vi "Beta Ver 1.0.vi"() -> ()   [LabVIEW 2015]
uses:
  <instrlib>/Keithley 622x LV 2009/Configure/Source/Typedefs/KE622x -- Current Range.ctl
  <instrlib>/Keithley 622x LV 2009/Configure/Source/Typedefs/KE622x -- Current Ranges.ctl
  <instrlib>/Keithley 622x LV 2009/Typedefs/KE622x -- On Off Control.ctl
  <instrlib>/Keithley 622x LV 2009/Utility/Typedefs/KE622x -- Instrument Type.ctl
  <instrlib>/Keithley 622x LV 2009/Configure/Source/Typedefs/KE622x -- Voltage Limit.ctl
  <instrlib>/Keithley 2000/Public/Configure/Configure DC Volts.vi
  <userlib>/LV-Link3/PolySubVIs/DtCreateAinChan.vi
  <userlib>/LV-Link3/PolySubVIs/DtOLReadMultipleSingle.vi
  <instrlib>/Keithley 2000/Keithley 2000.lvlib
  <instrlib>/Keithley 622x LV 2009/Keithley 622x.lvlib
panel:
  in  "Setup":u16(ring) items=["START, STOP, STEP, CONFIGURATION", "PRINCETON LOCK-IN AMP"]
  out "prev_time_const":i32
  out "prev_range":i32
  out "XTC":i32
  out "SEN":i32
  in  "Time Delay":u16(ring) items=["0.1", "1", "3", "10", "30", "60"]
  out "FILE":refnum<file>
  out "Tick":u32
  in  "MULTIPLE GRAPHS Y":u16(ring) items=["Linear", "Log"]
  in  "MULTIPLE GRAPHS X":u16(ring) items=["Linear", "Log"]
  in  "TIME GRAPH Y":u16(ring) items=["Linear", "Log"]
  in  "TIME GRAPH X":u16(ring) items=["Linear", "Log"]
  in  "Lock-In, Y":dbl=1.0
  in  "Lock-In, X":dbl=1.0
  in  "DAQ A4":dbl=1.0
  in  "DAQ A3":dbl=1.0
  in  "DAQ A2":dbl=1.0
  in  "DAQ A1":dbl=1.0
  in  "DAQ A0":dbl=1.0
  in  "2000":dbl=1.0
  in  "Current":dbl=1000.0
  in  "Display Type 3":u16(ring)=3 items=["X %", "Y %", "X Calibrated", "Y Calibrated", "Mag %", "Mag Calibrated", "Phase Degrees", "Ratio", "ADC 1", "ADC 2", "ADC 3", "ADC 4 ", "Noise %", "Noise Calibrated", "Ref Frequency", "", ""]
  in  "Display Type 2":u16(ring)=2 items=["X %", "Y %", "X Calibrated", "Y Calibrated", "Mag %", "Mag Calibrated", "Phase Degrees", "Ratio", "ADC 1", "ADC 2", "ADC 3", "ADC 4 ", "Noise %", "Noise Calibrated", "Ref Frequency", "", ""]
  out "Units 3":string
  out "Display 3":dbl format="%.3f"
  out "Units 2":string
  out "Display 2":dbl format="%.3f"
  out "DAQ A4":dbl format="%#_13g"
  out "DAQ_clust":T1
  out "DAQ A3":dbl format="%#_13g"
  out "DAQ A2":dbl format="%#_13g"
  out "DAQ A1":dbl format="%#_13g"
  out "Real stop cur":dbl format="%#_13g"
  out "Real start cur":dbl format="%#_13g"
  in  "Stop cur prefix":u16(ring)=2
  in  "Start cur prefix":u16(ring)=2
  out "MULTIPLE GRAPHS":cluster{dbl[], dbl[]}[](graph)
  in  "X-Axis":T2(ring)
  in  "Range":u8(ring)=20 items=["100nV", "200nV", "500nV", "1µV", "2µV", "5µV", "10µV", "20µV", "50µV", "100µV", "200µV", "500µV", "1mV", "2mV", "5mV", "10mV", "20mV", "50mV", "100mV", "200mV", "500mV", "1V"]
  in  "Display Type copy":u16(ring)=3 items=["X %", "Y %", "X Calibrated", "Y Calibrated", "Mag %", "Mag Calibrated", "Phase Degrees", "Ratio", "ADC 1", "ADC 2", "ADC 3", "ADC 4 ", "Noise %", "Noise Calibrated", "Ref Frequency", "", ""]
  out "Units copy":string
  out "Display copy":dbl format="%.3f"
  out "Overload":bool
  out "Display":dbl format="%.3f"
  out "Units":string
  in  "Display Type":u16(ring)=2 items=["X %", "Y %", "X Calibrated", "Y Calibrated", "Mag %", "Mag Calibrated", "Phase Degrees", "Ratio", "ADC 1", "ADC 2", "ADC 3", "ADC 4 ", "Noise %", "Noise Calibrated", "Ref Frequency", "", ""]
  in  "Time Constant":u16(ring)=7 items=["MIN", "1ms", "3ms", "10ms", "30ms", "100ms", "300ms", "1s", "3s", "10s", "30s", "100s", "300s"]
  in  "Slope":u8(ring) items=["6db/octave", "12dB/octave"]
  in  "Dynamic Reserve":u16(ring)=1 items=["High Stability", "Normal", "High Reserve"]
  in  "Auto Sensitivity":bool
  in  "Auto Measure":bool
  out "6221_error_out":errorcluster
  out "2000_error_out":errorcluster
  out "5110_error_out":errorcluster
  out "Input Mode":i32(ring) items=[" Voltage Input (A or A-B) ", "Current Input 10E6 V/A", "Current Input 10E8 V/A"]
  out "5110":refnum<visa-resource-name>
  in  "GPIB Address":i8=11 min=1 max=32 step=1
  out "DAQ A0":dbl format="%#_13g"
  out "2000":dbl format="%#_13g"
  in  "Device":string(combo)
  in  "Number \nof points":i32=10
  in  "Folder\nprename":string
  out "TIME GRAPH":cluster{dbl[], dbl[]}[](graph)
  out "T0":u32
  out "LIMIT":bool
  out "LIMIT":bool
  out "Error Code":string
  in  "Comments":string
  out "2000":refnum<visa-resource-name>
  out "6221":refnum<visa-resource-name>
  out "Step  (A)":dbl=5e-05 format="%#_3p"
  in  "Stop\ncurrent (A)":dbl=2.0 format="%#_6p"
  in  "Start \ncurrent (A)":dbl=1.0 format="%#_6p"
  in  "Check For SCPI Errors? (T)":bool=TRUE
  out "Interlock Tripped?":bool
  out "Compliance?":bool
  in  "Turn Off Output \nIf Compliance?":bool=TRUE
  in  "Turning ON/OFF\ncurrent output":T3=enum."On"
  in  "Range Selection":T4={"Auto Range?"=TRUE, "Man / Selected\nRange"=enum."2nA"}
  # "FILE CONFIGURATION"
  # "ADMIN PANEL"
  # "MULTIPLIERS"
  # "SCALES"
  # "KEITHLEY 6221 CONFIGURATION (ADMIN ONLY)"
  # "KEITHLEY DAQ CONFIGURATION (ADMIN ONLY)"
  # "PRINCETON LOCK-IN AMP (ADMIN ONLY)"
  # "I don't know what the hell it is,\njust don't touch it"
  # "INPUT CONFIGURATION"
  # "READINGS"
  # "IF ON"
  # "Compliance = Limiting output voltage\nThis switch determines if we want to switch \noff the current output if wee exceed compliance"
  # "SCALES"
  # "There is a safe switch at \nthe back of the instrument \nThis indicator shows if it is on"
  # "You have hit a damn jackpot \nby exceeding the limited voltage\nCongrats"
  # "LOCK-IN READINGS"
  # "RIGHT DISPLAY"
  # "LEFT DISPLAY"
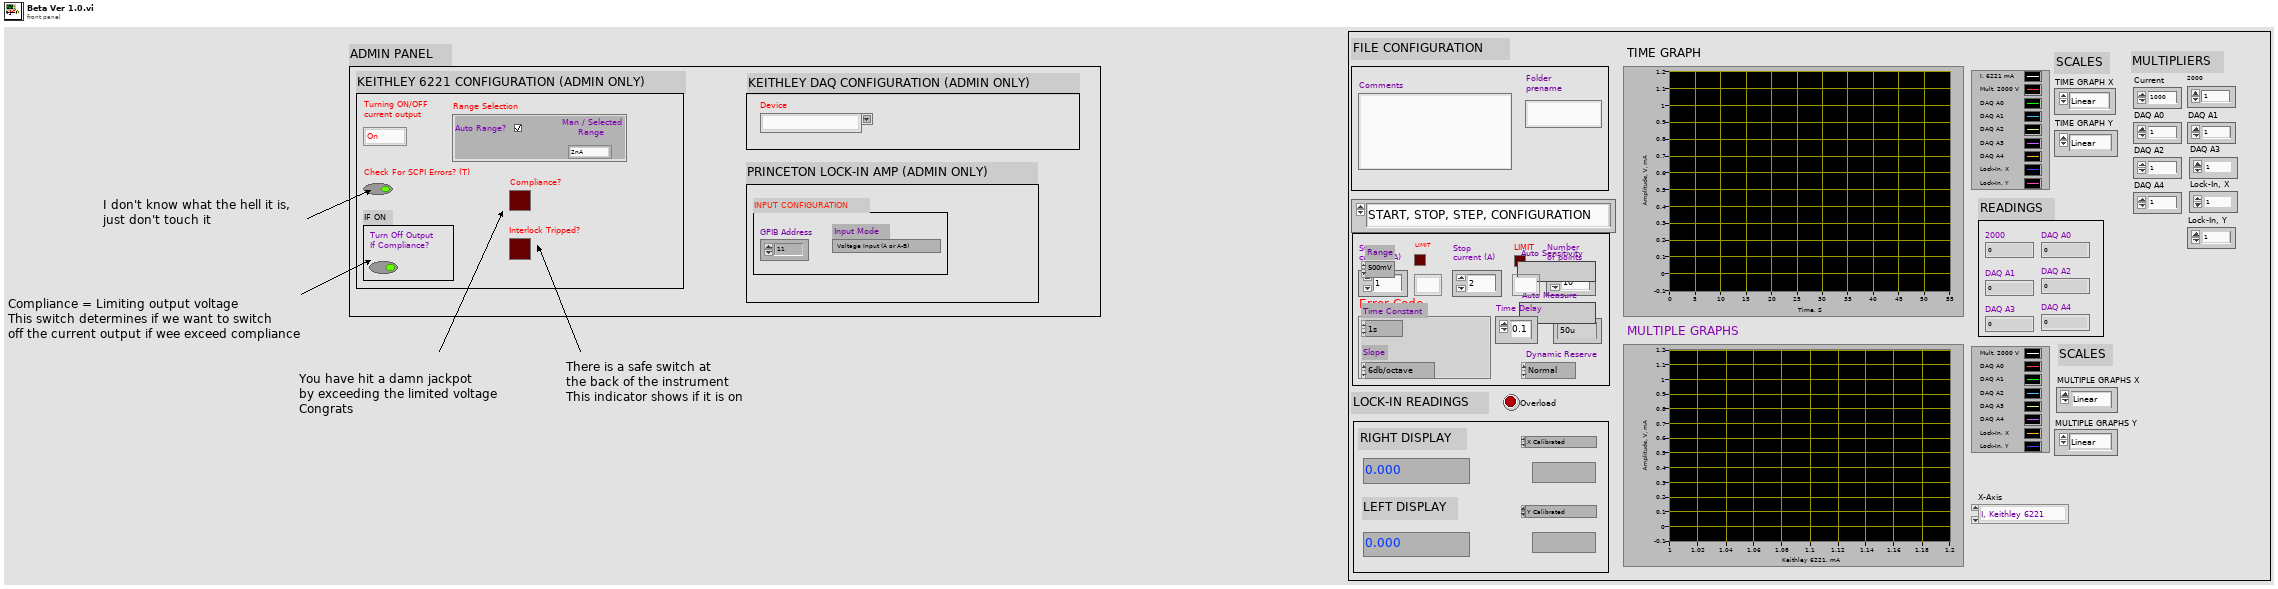
[diagram p1: front panel]
types:
  T1 = cluster{"Task out":i32, "Actual Number of Channels":u32, "error out":errorcluster}
  T2 = enum16{"I, Keithley 6221", "V, Keithley 2000", "V, Keithley DAQ A0", "V, Keithley DAQ A1", "V, Keithley DAQ A2", "V, Keithley DAQ A3", "V, Keithley DAQ A4", "V, Lock-In X", "V, Lock-In Y"}
  T3 = typedef "Keithley 622x.lvlib/KE622x -- On Off Control.ctl" = enum16{"Off", "On"}
  T4 = typedef "Keithley 622x.lvlib/KE622x -- Current Range.ctl" = cluster{"Auto Range?":bool, "Man / Selected\nRange":T5}
  T5 = typedef "Keithley 622x.lvlib/KE622x -- Current Ranges.ctl" = enum16{"2nA", "20nA", "200nA", "2uA", "20uA", "200uA", "2mA", "20mA", "100mA"}
  T6 = typedef "Keithley 622x.lvlib/KE622x -- Instrument Type.ctl" = enum16{"KE6220", "KE6221"}
  T7 = typedef "Keithley 622x.lvlib/KE622x -- Voltage Limit.ctl" = dbl
  T8 = cluster{"Task out":i32, "error out":errorcluster}
  T9 = cluster{dbl, dbl, dbl, dbl, dbl, "Measurement":dbl}
  T10 = cluster{dbl[], dbl[], dbl[], dbl[], dbl[], dbl[], dbl[], dbl[], dbl[], dbl[]}
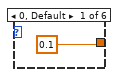
[diagram p2: hidden frame]
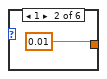
[diagram p3: hidden frame]
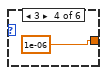
[diagram p4: hidden frame]
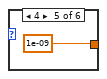
[diagram p5: hidden frame]
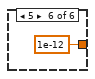
[diagram p6: hidden frame]
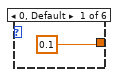
[diagram p7: hidden frame]
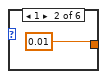
[diagram p8: hidden frame]
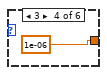
[diagram p9: hidden frame]
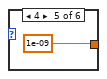
[diagram p10: hidden frame]
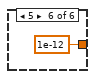
[diagram p11: hidden frame]
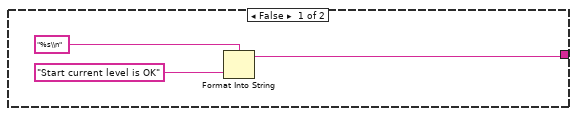
[diagram p12: hidden frame]
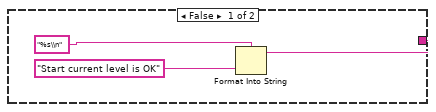
[diagram p13: hidden frame]
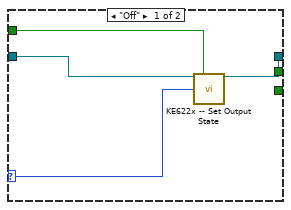
[diagram p14: hidden frame]
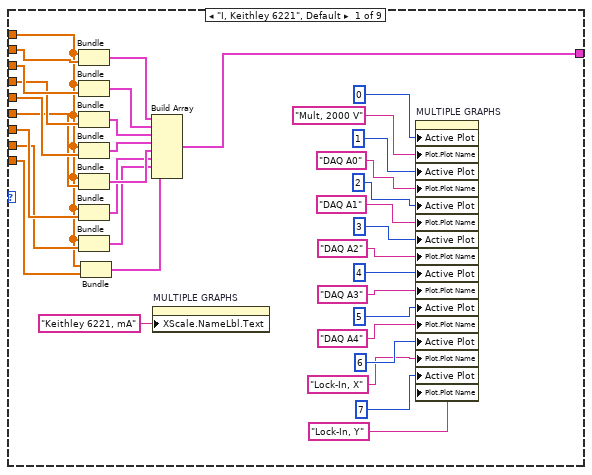
[diagram p15: hidden frame]
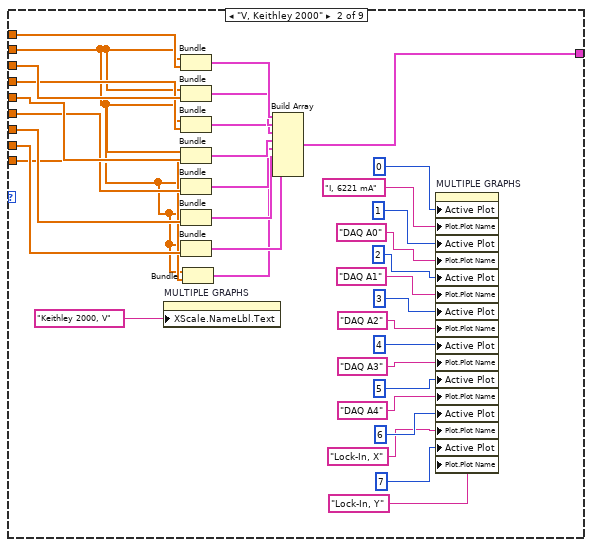
[diagram p16: hidden frame]
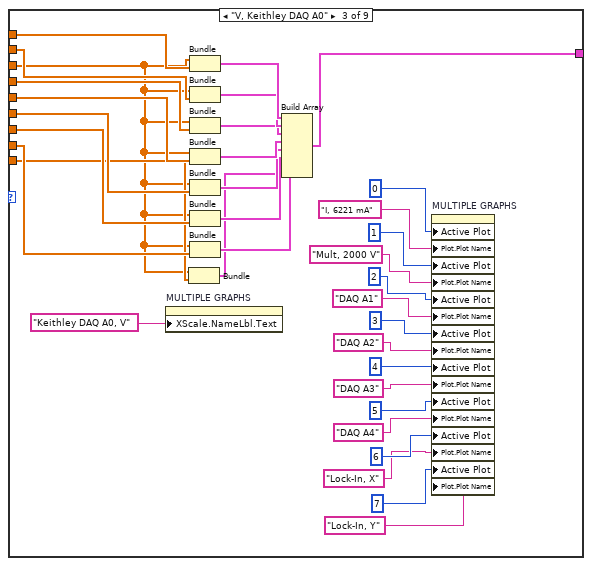
[diagram p17: hidden frame]
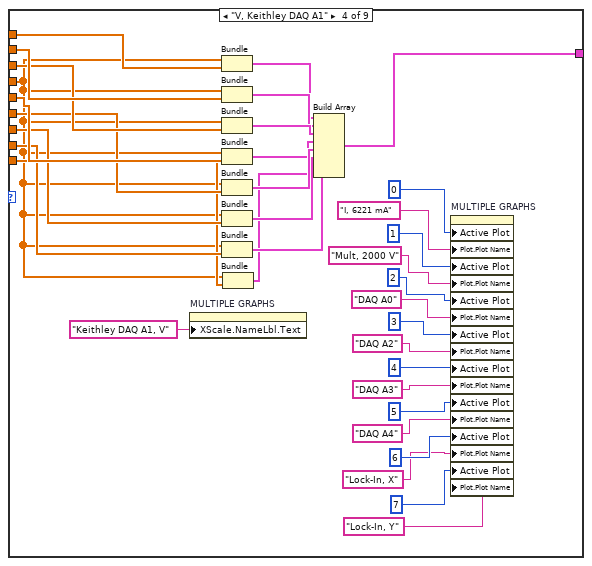
[diagram p18: hidden frame]
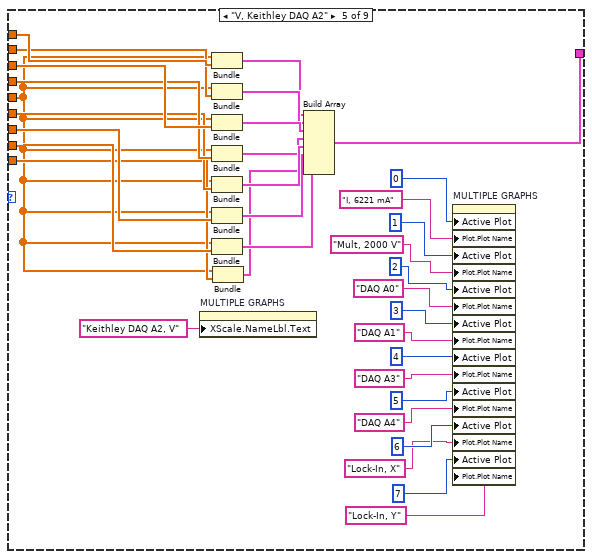
[diagram p19: hidden frame]
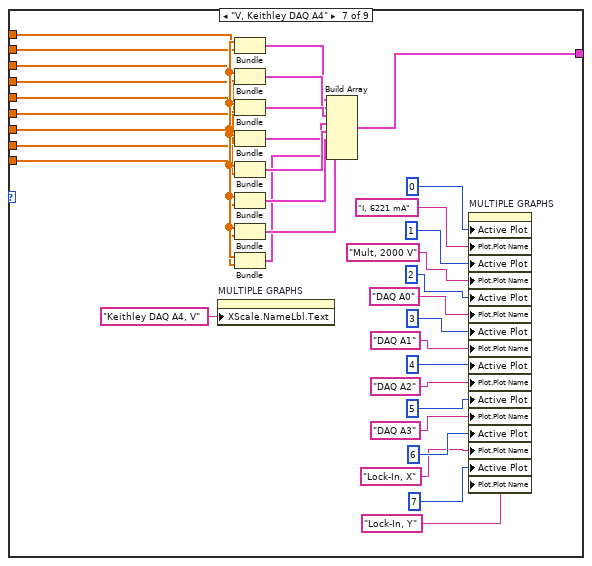
[diagram p20: hidden frame]
diagram:
  n1 = flat-sequence {
    tunnel: [w179] -> w7
    tunnel: [w178] -> w6
    tunnel: [w177] -> w5
    tunnel: [w176] -> w4
    tunnel: [w175] -> w3
    tunnel: [w174] -> w2
    tunnel: [w163] -> w1
    tunnel: w7 -> [w1070]
    tunnel: w6 -> [w1069]
    tunnel: w5 -> [w1068]
    tunnel: w4 -> [w1067]
    tunnel: w3 -> [w1066]
    tunnel: w2 -> [w1065]
    tunnel: w1 -> [w1064]
    frame #0 {
      # "File configuration"
      # "Start, Stop, Step"
      # "Initializing instruments"
      n2 = flat-sequence {
        frame #0 {
          w15 = TRUE  # reset
          w14 = FALSE  # ID query
          # "Initialize Lock-In 5110"
          # "Initialize Keithley 2000"
          # "Initialize Keithley 6221"
          n3 = call <instrlib>:"Initialize.vi"("VISA resource name"=refnum<visa-resource-name> "KEITHLEY_MULTIMETER") -> ("VISA resource name out"=w19:refnum<visa-resource-name>)  [unwired: 17 in, 1 out]
          n4 = call <instrlib>:"Initialize.vi"("VISA resource name"=refnum<visa-resource-name> "KEITHLEY_DC_AC_CURRENT_SOURCE", "Error Queue Option"=enum16{"Clear Error Queue", "Error Query"}."Clear Error Queue", "Instrument Type"=KE622x_--_Instrument_Type."KE6221") -> ("VISA resource name out"=→"6221":refnum<visa-resource-name>, "error out"=→"6221_error_out":errorcluster)  [unwired: 11 in]
          n5 = call "SR51XX Initialize"("VISA session (for class)"=refnum<visa-resource-name> "LOCK_IN_5110_PRINCETON", "Interface"=FALSE, "ID query"=w14, "GPIB Address"="GPIB Address", "reset"=w15) -> ("VISA session"=→"5110":refnum<visa-resource-name>, "error out"=→"5110_error_out":errorcluster)  [unwired: 8 in, 1 out]
          n6 = call-poly <instrlib>:"Configure Measurement.vi"("VISA resource name"=w19) -> ("VISA resource name out"=→"2000":refnum<visa-resource-name>, "error out"=→"2000_error_out":errorcluster)  [unwired: 17 in]
        }
        frame #1 {
          # "Initialize Keithley DAQ \n(getting board name)"
          n7 = call <userlib>:"DtOLGetBoardNames.vi"() -> ("Number of boards"=w24:u32)  [unwired: 9 in, 2 out]
          n8 = Initialize Array("", w24) -> (w26:string[])
          n9 = for {
            N: w24 -> [_]
            shift-right: [w32] -> w29
            shift-left: w26 -> [w33]
            i -> [w31]
            n10 = Add(x=1, y=w31) -> (x+y=w35:i32)
            n11 = call <userlib>:"DtOLGetBoardNames.vi"("Select Board"=w35) -> ("Board Name"=w30:string)  [unwired: 8 in, 2 out]
            n12 = Replace Array Subset(array=w33, new element=w30, index=w31) -> (w32:string[])
          }
          n13 = Index Array(array=w29, index=0) -> (element=w28:string)
          n14 = property on="Device" class="CmbBox"("Strings[]"=w29, "Value"=w28) -> ()  [unwired: 2 in, 2 out]
        }
        frame #2 {
          # "Putting in a loop \ninstead of \"STOP\""
          n15 = case shown="2" "Start cur prefix" {
            tunnel: [0.1 0.01 0.001 1e-06 1e-09 1e-12] -> w41
            frame 0, Default {
            }
            frame 1 {
            }
            frame 2 {
            }
            frame 3 {
            }
            frame 4 {
            }
            frame 5 {
            }
          }
          n16 = case shown="2" "Stop cur prefix" {
            tunnel: [0.1 0.01 0.001 1e-06 1e-09 1e-12] -> w39
            frame 0, Default {
            }
            frame 1 {
            }
            frame 2 {
            }
            frame 3 {
            }
            frame 4 {
            }
            frame 5 {
            }
          }
          n17 = Multiply(x=w41, y="Start \ncurrent (A)") -> (x*y=w37:dbl)
          "Real start cur" <- w37
          n18 = Multiply(x=w39, y="Stop\ncurrent (A)") -> (x*y=w36:dbl)
          "Real stop cur" <- w36
          n19 = Greater?(x=w36, y=T7 0.01) -> (0:w47:bool)
          n20 = Greater?(x=w37, y=T7 0.01) -> (0:w46:bool)
          n21 = case shown="True" w47 {
            selector: w47 -> [_ w66]
            tunnel: [w63 w69] -> w49
            frame False {
              n22 = Format Into String(format string="%s\\n", "Start current level is OK" ("false string")) -> (resulting string=w63:string)  [unwired: 2 in, 1 out]
            }
            frame True {
              n23 = flat-sequence {
                tunnel: [w71] -> w68
                tunnel: [w70] -> w67
                tunnel: w66 -> [w70]
                tunnel: [w75] -> w69
                tunnel: w68 -> [w75]
                tunnel: w67 -> [w76]
                frame #0 {
                  n24 = Format Into String(format string="%s\\n%s\\n", "Stop current level" ("String"), "exceeded the  limit: 10mA" ("input 2")) -> (resulting string=w71:string)  [unwired: 2 in, 1 out]
                }
                frame #1 {
                  n25 = while {
                    tunnel: w76 -> [w77]
                    stop <- w77 continue-if-true
                    "LIMIT" <- w77
                  }
                  n26 = property on="Error Code" class="Str"("Text.Text"=w75) -> ()  [unwired: 2 in, 2 out]
                }
              }
            }
          }
          n27 = case shown="True" w46 {
            selector: w46 -> [_ w82]
            tunnel: [w78 w84] -> w48
            frame False {
              n28 = Format Into String(format string="%s\\n", "Start current level is OK" ("false string")) -> (resulting string=w78:string)  [unwired: 2 in, 1 out]
            }
            frame True {
              n29 = flat-sequence {
                tunnel: [w86] -> w83
                tunnel: w82 -> [w85]
                tunnel: [w85] -> w81
                tunnel: [w90] -> w84
                tunnel: w83 -> [w90]
                tunnel: w81 -> [w91]
                frame #0 {
                  n30 = Format Into String(format string="%s\\n%s\\n", "Start current level" ("String"), "exceeded the limit: 10mA" ("input 2")) -> (resulting string=w86:string)  [unwired: 2 in, 1 out]
                }
                frame #1 {
                  n31 = while {
                    tunnel: w91 -> [w92]
                    stop <- w92 continue-if-true
                    "LIMIT" <- w92
                  }
                  n32 = property on="Error Code" class="Str"("Text.Text"=w90) -> ()  [unwired: 2 in, 2 out]
                }
              }
            }
          }
          n33 = Concatenate Strings(w48, w49) -> (→"Error Code":string)
        }
        frame #3 {
          # "Calculating steps by number\nof points"
          n34 = local read "Real stop cur"() -> (w96:dbl)
          n35 = local read "Real start cur"() -> (w95:dbl)
          n36 = Subtract(x=w96, y=w95) -> (x-y=w93:dbl)
          n37 = Divide(x=w93, y="Number \nof points") -> (x/y=→"Step  (A)":dbl)
        }
        frame #4 {
          # "Adding headlines"
          # "Creating folder&file"
          # "Creating comments"
          # "Writing instr params"
          n38 = local read "5110"() -> (w110:refnum<visa-resource-name>)
          n39 = local read "Real stop cur"() -> (w112:dbl)
          n40 = local read "Real start cur"() -> (w111:dbl)
          n41 = call "folder_creation.vi"("Name"="Folder\nprename") -> ("String"=w119:string)
          n42 = call "file_creation.vi"("String"=w119) -> ("refnum out"=w113:refnum<file>)
          "FILE" <- w113
          n43 = call "com_inst.vi"("Stop current"=w112, "Start current"=w111, "VISA session (for class)"=w110) -> ("XTC"=w108:i32, "SEN"=w109:i32, "concatenated string"=w107:string)
          "SEN" <- w109
          "XTC" <- w108
          n44 = Format Into String(format string="# %s\\n", initial string=w113, "Comments") -> (resulting string=w115:refnum<file>)  [unwired: 1 in, 1 out]
          n45 = property on="Time Constant" class="Ring (strict)"("Value"=w108) -> ()  [unwired: 2 in, 2 out]
          n46 = Format Into String(format string="# %s\\n", initial string=w115, w107) -> (resulting string=w114:refnum<file>)  [unwired: 1 in, 1 out]
          n47 = property on="Range" class="Ring (strict)"("Value"=w109) -> ()  [unwired: 2 in, 2 out]
          n48 = Format Into String(format string="# %-6s  %-12s %-12s %-14s %-12s %-14s %-12s %-12s %-14s%-14s\\n", initial string=w114, "t, ms" ("input 3"), "6221, A" ("input 3"), "2000, V" ("input 1"), "5110_X, V" ("input 3"), "5110_Y, V " ("input 3"), "DAQ A0, V" ("input 2"), "DAQ A1, V" ("input 2"), "DAQ A2, V" ("input 2"), "DAQ A3, V" ("input 2"), "DAQ A4, V" ("input 2")) -> ()  [unwired: 1 in, 2 out]
        }
        frame #5 {
          # "Variables"
          # "Time Intit"
          n49 = property on="SEN" class="DigNum (strict)"() -> ("Value"=→"prev_range":i32)  [unwired: 2 in, 2 out]
          n50 = property on="XTC" class="DigNum (strict)"() -> ("Value"=→"prev_time_const":i32)  [unwired: 2 in, 2 out]
          n51 = Wait Until Next ms Multiple(millisecond multiple=u32 1000) -> (millisecond timer value=→"T0":u32)
        }
      }
    }
    frame #1 {
      # "Configuring Keithley DAQ just before measuments"
      # "Configuring Keithley 6221 just before measuments"
      n52 = flat-sequence {
        tunnel: [w137] -> w127
        tunnel: [w155] -> _
        tunnel: [w157] -> _
        tunnel: w127 -> [w156]
        frame #0 {
          # "Current range \nselection check"
          # "Checking for compliance\nand interlock errors"
          n53 = local read "6221"() -> (w140:refnum<visa-resource-name>)
          n54 = call <instrlib>:"KE622x -- Set Current Range.vi"("Resource In"=w140, "Current Range In"="Range Selection", "Read Back Set Values? (T)"=FALSE) -> ("Resource Out (dupl)"=w145:refnum<visa-resource-name>)  [unwired: 10 in, 2 out]
          n55 = case shown="\"On\"" "Turning ON/OFF\ncurrent output" {
            selector: "Turning ON/OFF\ncurrent output" -> [w149 _]
            tunnel: [_ w153] -> w143
            tunnel: [_ w152] -> w144
            tunnel: "Check For SCPI Errors? (T)" -> [w148 _]
            tunnel: w145 -> [w146 w151]
            tunnel: [w147 w150] -> w137
            frame "Off" {
              n56 = call <instrlib>:"KE622x -- Set Output State.vi"("Resource In"=w146, "Check For SCPI Errors? (T)"=w148, "Output State"=w149) -> ("Resource Out (dupl)"=w147:refnum<visa-resource-name>)  [unwired: 11 in, 1 out]
            }
            frame "On" {
              n57 = call <instrlib>:"KE622x -- Turn Output On And Check For Errors.vi"("Resource In"=w151, "Turn Off Output If Compliance?"="Turn Off Output \nIf Compliance?") -> ("Resource Out (dupl)"=w150:refnum<visa-resource-name>, "Interlock Tripped?"=w153:bool, "Compliance?"=w152:bool)  [unwired: 10 in, 1 out]
            }
          }
          "Interlock Tripped?" <- w143
          "Compliance?" <- w144
        }
        frame #1 {
          # "Setting start current"
          n58 = local read "Real start cur"() -> (w155:dbl)
          n59 = Wait (ms)(milliseconds to wait=u32 100) -> ()  [unwired: 1 out]
          n60 = call <instrlib>:"KE622x -- Set Current Level.vi"("Resource In"=w156, "Current Level (A) In"=w155) -> ("Resource Out (dupl)"=w157:refnum<visa-resource-name>)  [unwired: 12 in, 1 out]
        }
      }
      n61 = flat-sequence {
        frame #0 {
          w132 = 100 items=["SingleEnded"=100, "Differential"=101] ("Channel Type")
          # "Configure the input channel"
          n62 = call-poly <userlib>:"DtOLCreateTask.vi"("Channel Type"=w132, "Range Min"=-10.0, "Range Max"=10.0, "Board Name"="Device", "Channel"="0:4" ("Channels")) -> ("Task out"=w131:i32, "Actual Number of Channels"=w130:u32, "error out"=w129:errorcluster)  [unwired: 8 in]
          n63 = Bundle("Task out"=w131, "Actual Number of Channels"=w130, "error out"=w129) -> (→"DAQ_clust":T1)  [unwired: 1 in]
        }
      }
    }
    frame #2 {
      n64 = local read "5110"() -> (w170:refnum<visa-resource-name>)
      n65 = local read "2000"() -> (w169:refnum<visa-resource-name>)
      n66 = local read "6221"() -> (w168:refnum<visa-resource-name>)
      n67 = local read "5110_error_out"() -> (w167:errorcluster)
      n68 = local read "6221_error_out"() -> (w166:errorcluster)
      n69 = local read "2000_error_out"() -> (w165:errorcluster)
      n70 = local read "DAQ_clust"() -> (w164:T1)
      n71 = while {
        shift-right: [w366] -> _
        shift-left: dbl[] [] -> [w467]
        shift-right: [w367] -> _
        shift-left: i32[] [] -> [w466]
        tunnel: w169 -> [w464]
        tunnel: w168 -> [w463]
        shift-right: [w338] -> _
        shift-left: dbl[] [] -> [w457]
        tunnel: [w456] -> w179
        tunnel: [w455] -> w178
        tunnel: [w453] -> w177
        tunnel: [w451] -> w176
        tunnel: w170 -> [w449]
        tunnel: w167 -> [w448]
        tunnel: w166 -> [w440]
        tunnel: w165 -> [w439]
        tunnel: [w414] -> w175
        tunnel: [w412] -> w174
        shift-right: [w340] -> _
        shift-left: dbl[] [] -> [w411]
        shift-right: [w341] -> _
        shift-left: dbl[] [] -> [w410]
        shift-right: [w368] -> _
        shift-left: dbl[] [] -> [w407]
        tunnel: w164 -> [w381]
        tunnel: [w380] -> w163
        shift-right: [w365] -> _
        shift-left: dbl[] [] -> [w379]
        shift-right: [w364] -> _
        shift-left: dbl[] [] -> [w378]
        shift-right: [w363] -> _
        shift-left: dbl[] [] -> [w377]
        shift-right: [w339] -> _
        shift-left: dbl[] [] -> [w343]
        i -> [w441]
        stop <- w458 stop-if-true
        # "V, DAQ A4"
        # "V, DAQ A3"
        # "V, DAQ A2"
        # "V, DAQ A1"
        # "Y-V, 5110"
        # "X-V, 5110"
        # "I, 6221"
        # "Config delay"
        # "Control subVI 5110"
        # "Read config 5110"
        # "Measurement config 5110"
        # "Time config 5110"
        # "Configuring Right Display 5110"
        # "Configuring Left Display 5110"
        # "Setting 6221 current"
        # "Delay before measuremens"
        # "Getting the data from DAQ and 2000"
        # "Changing input current"
        # "Time"
        # "V, DAQ A0"
        # "V, 2000"
        n72 = local read "T0"() -> (w465:u32)
        n73 = Quotient & Remainder(x=w441, y=10) -> (floor(x/y)=w446:i32)  [unwired: 1 out]
        n74 = Equal?(x=0, y=w441) -> (x = y?=w443:bool)
        n75 = Subtract(x=w432, y=w465) -> (x-y=w388:u32)
        n76 = Equal?(x=1, y=w446) -> (x = y?=w442:bool)
        n77 = flat-sequence {
          tunnel: w464 -> [w792]
          tunnel: [w792] -> w406
          tunnel: w463 -> [w791]
          tunnel: [w791] -> w404
          tunnel: w449 -> [w790]
          tunnel: [w790] -> w402
          tunnel: [w789] -> w400
          tunnel: w448 -> [w789]
          tunnel: w443 -> [w788]
          tunnel: [w788] -> w398
          tunnel: w442 -> [w787]
          tunnel: [w787] -> w396
          tunnel: w440 -> [w786]
          tunnel: [w786] -> w394
          tunnel: w439 -> [w785]
          tunnel: [w785] -> w392
          tunnel: [w783] -> w432
          tunnel: [w784] -> w382
          tunnel: w381 -> [w784]
          tunnel: w406 -> [w802]
          tunnel: [w802] -> w405
          tunnel: w404 -> [w801]
          tunnel: [w801] -> w403
          tunnel: w402 -> [w800]
          tunnel: [w800] -> w401
          tunnel: w400 -> [w799]
          tunnel: [w799] -> w399
          tunnel: w398 -> [w798]
          tunnel: [w798] -> w397
          tunnel: w396 -> [w797]
          tunnel: [w797] -> w395
          tunnel: w394 -> [w796]
          tunnel: [w796] -> w393
          tunnel: w392 -> [w795]
          tunnel: [w795] -> w391
          tunnel: [w794] -> w383
          tunnel: w382 -> [w794]
          tunnel: w405 -> [w819]
          tunnel: [w819] -> w431
          tunnel: w403 -> [w818]
          tunnel: [w818] -> w430
          tunnel: w401 -> [w817]
          tunnel: w399 -> [w814]
          tunnel: [w813] -> w429
          tunnel: [w812] -> w428
          tunnel: w397 -> [w811]
          tunnel: [w811] -> w427
          tunnel: w395 -> [w810]
          tunnel: w393 -> [w809]
          tunnel: [w809] -> w426
          tunnel: w391 -> [w808]
          tunnel: [w808] -> w425
          tunnel: [w807] -> w384
          tunnel: w383 -> [w807]
          tunnel: w431 -> [w844]
          tunnel: [w844] -> w239
          tunnel: w430 -> [w843]
          tunnel: [w843] -> w237
          tunnel: w429 -> [w840]
          tunnel: [w839] -> w235
          tunnel: w428 -> [w838]
          tunnel: [w837] -> w233
          tunnel: w427 -> [w835]
          tunnel: [w835] -> w231
          tunnel: w426 -> [w842]
          tunnel: [w842] -> w229
          tunnel: w425 -> [w841]
          tunnel: [w841] -> w227
          tunnel: ["Auto Measure"] -> w225
          tunnel: ["Auto Sensitivity"] -> w223
          tunnel: [w830] -> w221
          tunnel: [w828] -> w219
          tunnel: w384 -> [w828]
          tunnel: w239 -> [w858]
          tunnel: [w858] -> w238
          tunnel: w237 -> [w857]
          tunnel: [w857] -> w236
          tunnel: w235 -> [w845]
          tunnel: [w845] -> w234
          tunnel: w233 -> [w856]
          tunnel: [w856] -> w232
          tunnel: w231 -> [w855]
          tunnel: [w855] -> w230
          tunnel: w229 -> [w854]
          tunnel: [w854] -> w228
          tunnel: w227 -> [w853]
          tunnel: [w853] -> w226
          tunnel: w225 -> [w852]
          tunnel: [w852] -> w224
          tunnel: w223 -> [w851]
          tunnel: [w851] -> w222
          tunnel: w221 -> [w850]
          tunnel: [w850] -> w220
          tunnel: w219 -> [w849]
          tunnel: [w849] -> w218
          tunnel: w238 -> [w885]
          tunnel: [w885] -> w195
          tunnel: w236 -> [w884]
          tunnel: [w884] -> w197
          tunnel: w234 -> [w877]
          tunnel: w232 -> [w875]
          tunnel: [w874] -> w199
          tunnel: w230 -> [w881]
          tunnel: [w881] -> w201
          tunnel: w228 -> [w883]
          tunnel: [w883] -> w203
          tunnel: w226 -> [w882]
          tunnel: [w882] -> w205
          tunnel: w224 -> [w879]
          tunnel: [w879] -> w207
          tunnel: w222 -> [w880]
          tunnel: [w880] -> w209
          tunnel: w220 -> [w870]
          tunnel: [w870] -> w211
          tunnel: [w876] -> w213
          tunnel: ["Time Constant"] -> w215
          tunnel: ["Slope"] -> w217
          tunnel: [w868] -> w193
          tunnel: w218 -> [w868]
          tunnel: w217 -> [w901]
          tunnel: [w901] -> w216
          tunnel: w215 -> [w900]
          tunnel: [w900] -> w214
          tunnel: w213 -> [w888]
          tunnel: [w888] -> w212
          tunnel: w211 -> [w899]
          tunnel: [w899] -> w210
          tunnel: w209 -> [w898]
          tunnel: [w898] -> w208
          tunnel: w207 -> [w897]
          tunnel: [w897] -> w206
          tunnel: w205 -> [w896]
          tunnel: [w896] -> w204
          tunnel: w203 -> [w895]
          tunnel: [w895] -> w202
          tunnel: w201 -> [w894]
          tunnel: [w894] -> w200
          tunnel: w199 -> [w890]
          tunnel: [w890] -> w198
          tunnel: w197 -> [w893]
          tunnel: [w893] -> w196
          tunnel: w195 -> [w892]
          tunnel: [w892] -> w194
          tunnel: w193 -> [w891]
          tunnel: [w891] -> w192
          tunnel: [w931] -> w336
          tunnel: [w930] -> w335
          tunnel: [w916] -> w334
          tunnel: [w929] -> w333
          tunnel: [w928] -> w332
          tunnel: [w927] -> w331
          tunnel: [w926] -> w330
          tunnel: [w925] -> w329
          tunnel: [w918] -> w328
          tunnel: [w921] -> w327
          tunnel: [w919] -> w326
          tunnel: [w924] -> w325
          tunnel: w216 -> [w924]
          tunnel: w214 -> [w919]
          tunnel: w212 -> [w922]
          tunnel: w210 -> [w918]
          tunnel: w208 -> [w925]
          tunnel: w206 -> [w926]
          tunnel: w204 -> [w927]
          tunnel: w202 -> [w928]
          tunnel: w200 -> [w929]
          tunnel: w198 -> [w917]
          tunnel: w196 -> [w930]
          tunnel: w194 -> [w931]
          tunnel: [w910] -> w324
          tunnel: w192 -> [w910]
          tunnel: w336 -> [w954]
          tunnel: [w954] -> w323
          tunnel: w335 -> [w953]
          tunnel: [w953] -> w321
          tunnel: w334 -> [w945]
          tunnel: [w944] -> w319
          tunnel: w333 -> [w952]
          tunnel: [w952] -> w317
          tunnel: w332 -> [w951]
          tunnel: [w951] -> w315
          tunnel: w331 -> [w950]
          tunnel: [w950] -> w313
          tunnel: w330 -> [w949]
          tunnel: [w949] -> w311
          tunnel: w329 -> [w948]
          tunnel: [w948] -> w309
          tunnel: w328 -> [w939]
          tunnel: [w939] -> w307
          tunnel: w327 -> [w946]
          tunnel: [w943] -> w305
          tunnel: w326 -> [w941]
          tunnel: [w941] -> w303
          tunnel: w325 -> [w938]
          tunnel: [w938] -> w301
          tunnel: w324 -> [w947]
          tunnel: [w947] -> w299
          tunnel: [w934] -> w296
          tunnel: w323 -> [w977]
          tunnel: [w977] -> w322
          tunnel: w321 -> [w976]
          tunnel: [w976] -> w320
          tunnel: w319 -> [w967]
          tunnel: [w966] -> w318
          tunnel: w317 -> [w975]
          tunnel: [w975] -> w316
          tunnel: w315 -> [w974]
          tunnel: [w974] -> w314
          tunnel: w313 -> [w973]
          tunnel: [w973] -> w312
          tunnel: w311 -> [w972]
          tunnel: [w972] -> w310
          tunnel: w309 -> [w971]
          tunnel: [w971] -> w308
          tunnel: w307 -> [w962]
          tunnel: [w962] -> w306
          tunnel: w305 -> [w969]
          tunnel: [w968] -> w304
          tunnel: w303 -> [w964]
          tunnel: [w964] -> w302
          tunnel: w301 -> [w961]
          tunnel: [w961] -> w300
          tunnel: w299 -> [w970]
          tunnel: [w970] -> w298
          tunnel: [w957] -> w297
          tunnel: w322 -> [w999]
          tunnel: [w999] -> w424
          tunnel: w320 -> [w998]
          tunnel: [w998] -> w423
          tunnel: w318 -> [w985]
          tunnel: w316 -> [w997]
          tunnel: [w997] -> w422
          tunnel: w314 -> [w996]
          tunnel: [w996] -> w421
          tunnel: w312 -> [w995]
          tunnel: [w995] -> w420
          tunnel: w310 -> [w994]
          tunnel: [w994] -> w419
          tunnel: w308 -> [w993]
          tunnel: [w993] -> w418
          tunnel: w306 -> [w986]
          tunnel: w304 -> [w983]
          tunnel: [w982] -> w417
          tunnel: w302 -> [w987]
          tunnel: w300 -> [w988]
          tunnel: [w984] -> w416
          tunnel: [w981] -> w415
          tunnel: [w978] -> w385
          tunnel: w298 -> [w978]
          tunnel: [w1003] -> w462
          tunnel: w441 -> [w1011]
          tunnel: [w1007] -> w458
          tunnel: [w1001] -> w460
          tunnel: [w1009] -> w459
          tunnel: [w1006] -> w438
          tunnel: [w1005] -> w437
          tunnel: [w1004] -> w436
          tunnel: [w1002] -> w435
          tunnel: [w1001] -> w376
          tunnel: w415 -> [_]
          tunnel: w416 -> [w1004]
          tunnel: w417 -> [w1002]
          tunnel: w418 -> [_]
          tunnel: w419 -> [_]
          tunnel: w420 -> [w1006]
          tunnel: w421 -> [w1005]
          tunnel: w422 -> [_]
          tunnel: w423 -> [w1009]
          tunnel: w424 -> [w1003]
          tunnel: [w1000] -> w386
          tunnel: w385 -> [w1000]
          tunnel: w462 -> [w1024]
          tunnel: [w1024] -> w461
          tunnel: w460 -> [w1023]
          tunnel: w459 -> [w1022]
          tunnel: [w1021] -> w454
          tunnel: [w1020] -> w452
          tunnel: w438 -> [w1018]
          tunnel: w437 -> [w1019]
          tunnel: w436 -> [w1016]
          tunnel: w435 -> [w1017]
          tunnel: [w1018] -> w434
          tunnel: [w1017] -> w433
          tunnel: [w1016] -> w413
          tunnel: [w1015] -> w387
          tunnel: w386 -> [w1015]
          tunnel: [w1052] -> w380
          tunnel: [w1053] -> w412
          tunnel: [w1054] -> w414
          tunnel: [w1061] -> w450
          tunnel: [w1055] -> w351
          tunnel: [w1056] -> w451
          tunnel: [w1057] -> w453
          tunnel: [w1058] -> w455
          tunnel: [w1059] -> w456
          tunnel: [w1060] -> w350
          tunnel: [w1061] -> w346
          tunnel: [w1051] -> w349
          tunnel: [w1050] -> w348
          tunnel: [w1049] -> w347
          tunnel: w461 -> [w1048]
          tunnel: w454 -> [w1057]
          tunnel: w452 -> [w1056]
          tunnel: w434 -> [w1047]
          tunnel: w433 -> [w1054]
          tunnel: w413 -> [w1053]
          tunnel: w387 -> [w1046]
          frame #0 {
            n78 = Tick Count (ms)() -> (millisecond timer value=w783:u32)
            "Tick" <- w783
          }
          frame #1 {
            n79 = case shown="1" "Setup" {
              frame 0, Default {
                n80 = flat-sequence {
                  frame #0 {
                    w803 = FALSE ("Visible")
                    n81 = property on="Slope" class="Ring (strict)"("Visible"=w803) -> ()  [unwired: 2 in, 2 out]
                    n82 = property on="Range" class="Ring (strict)"("Visible"=w803) -> ()  [unwired: 2 in, 2 out]
                    n83 = property on="Time Constant" class="Ring (strict)"("Visible"=w803) -> ()  [unwired: 2 in, 2 out]
                    n84 = property on="Dynamic Reserve" class="Ring (strict)"("Visible"=w803) -> ()  [unwired: 2 in, 2 out]
                    n85 = property on="Auto Sensitivity" class="Bool (strict)"("Visible"=w803) -> ()  [unwired: 2 in, 2 out]
                    n86 = property on="Auto Measure" class="Bool (strict)"("Visible"=w803) -> ()  [unwired: 2 in, 2 out]
                  }
                  frame #1 {
                    w804 = TRUE ("Visible")
                    n87 = property on="Start \ncurrent (A)" class="DigNum (strict)"("Visible"=w804) -> ()  [unwired: 2 in, 2 out]
                    n88 = property on="Stop\ncurrent (A)" class="DigNum (strict)"("Visible"=w804) -> ()  [unwired: 2 in, 2 out]
                    n89 = property on="LIMIT" class="Bool (strict)"("Visible"=w804) -> ()  [unwired: 2 in, 2 out]
                    n90 = property on="LIMIT" class="Bool (strict)"("Visible"=w804) -> ()  [unwired: 2 in, 2 out]
                    n91 = property on="Start cur prefix" class="Ring (strict)"("Visible"=w804) -> ()  [unwired: 2 in, 2 out]
                    n92 = property on="Stop cur prefix" class="Ring (strict)"("Visible"=w804) -> ()  [unwired: 2 in, 2 out]
                    n93 = property on="Step  (A)" class="DigNum (strict)"("Visible"=w804) -> ()  [unwired: 2 in, 2 out]
                    n94 = property on="Number \nof points" class="DigNum (strict)"("Visible"=w804) -> ()  [unwired: 2 in, 2 out]
                    n95 = property on="Time Delay" class="Ring (strict)"("Visible"=w804) -> ()  [unwired: 2 in, 2 out]
                    n96 = property on="Error Code" class="Str"("Visible"=w804) -> ()  [unwired: 2 in, 2 out]
                  }
                }
              }
              frame 1 {
                n97 = flat-sequence {
                  frame #0 {
                    w805 = TRUE ("Visible")
                    n98 = property on="Slope" class="Ring (strict)"("Visible"=w805) -> ()  [unwired: 2 in, 2 out]
                    n99 = property on="Range" class="Ring (strict)"("Visible"=w805) -> ()  [unwired: 2 in, 2 out]
                    n100 = property on="Time Constant" class="Ring (strict)"("Visible"=w805) -> ()  [unwired: 2 in, 2 out]
                    n101 = property on="Dynamic Reserve" class="Ring (strict)"("Visible"=w805) -> ()  [unwired: 2 in, 2 out]
                    n102 = property on="Auto Sensitivity" class="Bool (strict)"("Visible"=w805) -> ()  [unwired: 2 in, 2 out]
                    n103 = property on="Auto Measure" class="Bool (strict)"("Visible"=w805) -> ()  [unwired: 2 in, 2 out]
                  }
                  frame #1 {
                    w806 = FALSE ("Visible")
                    n104 = property on="Start \ncurrent (A)" class="DigNum (strict)"("Visible"=w806) -> ()  [unwired: 2 in, 2 out]
                    n105 = property on="Stop\ncurrent (A)" class="DigNum (strict)"("Visible"=w806) -> ()  [unwired: 2 in, 2 out]
                    n106 = property on="LIMIT" class="Bool (strict)"("Visible"=w806) -> ()  [unwired: 2 in, 2 out]
                    n107 = property on="LIMIT" class="Bool (strict)"("Visible"=w806) -> ()  [unwired: 2 in, 2 out]
                    n108 = property on="Start cur prefix" class="Ring (strict)"("Visible"=w806) -> ()  [unwired: 2 in, 2 out]
                    n109 = property on="Stop cur prefix" class="Ring (strict)"("Visible"=w806) -> ()  [unwired: 2 in, 2 out]
                    n110 = property on="Step  (A)" class="DigNum (strict)"("Visible"=w806) -> ()  [unwired: 2 in, 2 out]
                    n111 = property on="Number \nof points" class="DigNum (strict)"("Visible"=w806) -> ()  [unwired: 2 in, 2 out]
                    n112 = property on="Time Delay" class="Ring (strict)"("Visible"=w806) -> ()  [unwired: 2 in, 2 out]
                    n113 = property on="Error Code" class="Str"("Visible"=w806) -> ()  [unwired: 2 in, 2 out]
                  }
                }
              }
            }
          }
          frame #2 {
            n114 = case shown="False" w810 {
              tunnel: w817 -> [w821 w826]
              tunnel: [w820 w824] -> w816
              tunnel: [w821 w823] -> w815
              tunnel: w814 -> [w820 w822]
              frame False {
              }
              frame True {
                n115 = call "SR51XX Read Preamp Input Mode"("VISA session (for class)"=w826, "error in (no error)"=w822) -> ("VISA session"=w823:refnum<visa-resource-name>, "Input Mode"=w825:i32, "error out"=w824:errorcluster)  [unwired: 15 in]
                n116 = local write "Input Mode"(w825) -> ()
              }
            }
            n117 = call "SR51XX Configure Signal Channel Input"("VISA session (for class)"=w815, "error in (no error)"=w816, "Update"=w811) -> ("VISA session"=w813:refnum<visa-resource-name>, "error out"=w812:errorcluster)  [unwired: 15 in]
          }
          frame #3 {
            n118 = local read "Input Mode"() -> (w836:i32)
            n119 = call "SR51XX Configure Sensitivity"("VISA session (for class)"=w840, "Input Mode"=w836, "Range"="Range", "error in (no error)"=w838, "Auto Sensitivity"="Auto Sensitivity", "Auto Measure"="Auto Measure", "Update"=w835) -> ("Range Annotations Out[]"=w829:string[], "VISA session"=w839:refnum<visa-resource-name>, "Auto Sensitivity out"=w832:bool, "Auto Measure out"=w831:bool, "Range Out"=w830:u8, "error out"=w837:errorcluster)  [unwired: 7 in]
            n120 = property on="Range" class="Ring (strict)"("Strings []"=w829) -> ()  [unwired: 2 in, 2 out]
            n121 = local write "Auto Sensitivity"(w832) -> ()
            n122 = local write "Auto Measure"(w831) -> ()
            n123 = local write "Range"(w830) -> ()
          }
          frame #4 {
            n124 = property on="prev_range" class="DigNum (strict)"() -> ("Value"=w847:i32)  [unwired: 2 in, 2 out]
            n125 = property on="Range" class="Ring (strict)"() -> ("Value"=w846:u8)  [unwired: 2 in, 2 out]
            n126 = Equal?(x=w846, y=w847) -> (x = y?=w848:bool)
            n127 = case shown="False" w848 {
              tunnel: w845 -> [w859 _]
              frame False {
                n128 = flat-sequence {
                  tunnel: w859 -> [w861]
                  frame #0 {
                    n129 = property on="Range" class="Ring (strict)"() -> ("Value"=w860:u8)  [unwired: 2 in, 2 out]
                    n130 = property on="prev_range" class="DigNum (strict)"("Value"=w860) -> ()  [unwired: 2 in, 2 out]
                  }
                  frame #1 {
                    n131 = call "read_sense.vi"("VISA session (for class)"=w861) -> ("sense"=w863:string)
                    n132 = Concatenate Strings("Sensitivity: " ("string"), w863) -> (w862:string)
                    n133 = local read "FILE"() -> (w866:refnum<file>)
                    n134 = Format Into String(format string="# %-s\\n", initial string=w866, w862) -> ()  [unwired: 1 in, 2 out]
                  }
                }
              }
              frame True {
              }
            }
          }
          frame #5 {
            n135 = Or(x=w880, y=w879) -> (x .or. y?=w878:bool)
            n136 = call "SR51XX Configure Output Channels - Slope, TC and Dyn Reserve"("VISA session (for class)"=w877, "Time Constant"="Time Constant", "Slope"="Slope", "Check TC"=w878, "Dynamic Reserve"="Dynamic Reserve", "error in (no error)"=w875, "Range"=w870, "Update"=w881) -> ("VISA session"=w876:refnum<visa-resource-name>, "Slope Out"=w871:u8, "Time Constant Out"=w872:u16, "error out"=w874:errorcluster)  [unwired: 8 in]
            n137 = local write "Slope"(w871) -> ()
            n138 = local write "Time Constant"(w872) -> ()
          }
          frame #6 {
            n139 = property on="prev_time_const" class="DigNum (strict)"() -> ("Value"=w887:i32)  [unwired: 2 in, 2 out]
            n140 = property on="Time Constant" class="Ring (strict)"() -> ("Value"=w886:u16)  [unwired: 2 in, 2 out]
            n141 = Equal?(x=w886, y=w887) -> (x = y?=w889:bool)
            n142 = case shown="False" w889 {
              tunnel: w888 -> [w902 _]
              frame False {
                n143 = flat-sequence {
                  tunnel: w902 -> [w904]
                  frame #0 {
                    n144 = property on="Time Constant" class="Ring (strict)"() -> ("Value"=w903:u16)  [unwired: 2 in, 2 out]
                    n145 = property on="prev_time_const" class="DigNum (strict)"("Value"=w903) -> ()  [unwired: 2 in, 2 out]
                  }
                  frame #1 {
                    n146 = call "read_time_const.vi"("VISA session (for class)"=w904) -> ("time_const"=w905:string)
                    n147 = Concatenate Strings("Time Constant: " ("string"), w905) -> (w906:string)
                    n148 = local read "FILE"() -> (w909:refnum<file>)
                    n149 = Format Into String(format string="# %-s\\n", initial string=w909, w906) -> ()  [unwired: 1 in, 2 out]
                  }
                }
              }
              frame True {
              }
            }
          }
          frame #7 {
            n150 = local read "Input Mode"() -> (w923:i32)
            n151 = call "SR5110 Read Output"("VISA session (for class)"=w922, "Input Mode"=w923, "Time Constant"=w919, "Display Type"="Display Type", "Range"=w918, "error in (no error)"=w917, "Slope"=w924) -> ("Units"=→"Units":string, "Display Precision"=w915:i32, "Display"=→"Display":dbl, "VISA session"=w921:refnum<visa-resource-name>, "Available Display Types Out"=w914:string[], "Overload"=→"Overload":bool, "error out"=w916:errorcluster)  [unwired: 4 in, 2 out]
            n152 = property on="Display Type" class="Ring (strict)"("Strings []"=w914) -> ()  [unwired: 2 in, 2 out]
            n153 = property on="Display" class="DigNum (strict)"("Precision"=w915) -> ()  [unwired: 2 in, 2 out]
          }
          frame #8 {
            n154 = local read "Input Mode"() -> (w942:i32)
            n155 = call "SR5110 Read Output"("VISA session (for class)"=w946, "Input Mode"=w942, "Time Constant"=w941, "Display Type"="Display Type 2", "Range"=w939, "error in (no error)"=w945, "Slope"=w938) -> ("Units"=w932:string, "Display Precision"=w936:i32, "Display"=w933:dbl, "VISA session"=w943:refnum<visa-resource-name>, "Available Display Types Out"=w937:string[], "error out"=w944:errorcluster)  [unwired: 4 in, 3 out]
            "Display 2" <- w933
            "Units 2" <- w932
            n156 = call "pref_to_num.vi"("string"=w932) -> ("Numeric"=w935:dbl)
            n157 = property on="Display Type 2" class="Ring (strict)"("Strings []"=w937) -> ()  [unwired: 2 in, 2 out]
            n158 = property on="Display 2" class="DigNum (strict)"("Precision"=w936) -> ()  [unwired: 2 in, 2 out]
            n159 = Multiply(x=w935, y=w933) -> (x*y=w934:dbl)
          }
          frame #9 {
            n160 = local read "Input Mode"() -> (w965:i32)
            n161 = call "SR5110 Read Output"("VISA session (for class)"=w969, "Input Mode"=w965, "Time Constant"=w964, "Display Type"="Display Type 3", "Range"=w962, "error in (no error)"=w967, "Slope"=w961) -> ("Units"=w956:string, "Display Precision"=w960:i32, "Display"=w955:dbl, "VISA session"=w968:refnum<visa-resource-name>, "Available Display Types Out"=w959:string[], "error out"=w966:errorcluster)  [unwired: 4 in, 3 out]
            "Display 3" <- w955
            "Units 3" <- w956
            n162 = property on="Display 3" class="DigNum (strict)"("Precision"=w960) -> ()  [unwired: 2 in, 2 out]
            n163 = call "pref_to_num.vi"("string"=w956) -> ("Numeric"=w958:dbl)
            n164 = property on="Display Type 3" class="Ring (strict)"("Strings []"=w959) -> ()  [unwired: 2 in, 2 out]
            n165 = Multiply(x=w958, y=w955) -> (x*y=w957:dbl)
          }
          frame #10 {
            n166 = local read "Input Mode"() -> (w992:i32)
            n167 = call "SR5110 Read Output"("VISA session (for class)"=w983, "Input Mode"=w992, "Time Constant"=w987, "Display Type"="Display Type copy", "Range"=w986, "error in (no error)"=w985, "Slope"=w988) -> ("Units"=→"Units copy":string, "Display Precision"=w989:i32, "Display"=→"Display copy":dbl, "VISA session"=w982:refnum<visa-resource-name>, "Reference Unlock"=w981:bool, "Available Display Types Out"=w990:string[], "error out"=w984:errorcluster)  [unwired: 4 in, 2 out]
            n168 = property on="Display Type copy" class="Ring (strict)"("Strings []"=w990) -> ()  [unwired: 2 in, 2 out]
            n169 = property on="Display copy" class="DigNum (strict)"("Precision"=w989) -> ()  [unwired: 2 in, 2 out]
          }
          frame #11 {
            n170 = local read "Step  (A)"() -> (w1012:dbl)
            n171 = local read "Real start cur"() -> (w1013:dbl)
            n172 = Multiply(x=w1012, y=w1011) -> (x*y=w1010:dbl)
            n173 = Add(x=w1013, y=w1010) -> (x+y=w1001:dbl)
            n174 = local read "Real stop cur"() -> (w1008:dbl)
            n175 = Greater Or Equal?(x=w1001, y=w1008) -> (x >= y?=w1007:bool)
          }
          frame #12 {
            n176 = call <instrlib>:"KE622x -- Set Current Level.vi"("Resource In"=w1022, "Current Level (A) In"=w1023, "error in (no error)"=w1019) -> ("Resource Out (dupl)"=w1020:refnum<visa-resource-name>, "error out"=w1021:errorcluster)  [unwired: 11 in]
            n177 = Wait Until Next ms Multiple(millisecond multiple=u32 50) -> ()  [unwired: 1 out]
          }
          frame #13 {
            n178 = Unbundle(w1046) -> ("Task out"=w1045:i32, "Actual Number of Channels"=w1043:u32, "error out"=w1044:errorcluster)
            n179 = call <instrlib>:"Data Read Single.vi"("VISA resource name"=w1048, "error in (no error)"=w1047) -> ("VISA resource name out"=w1058:refnum<visa-resource-name>, "Measurement"=w1061:dbl, "error out"=w1059:errorcluster)  [unwired: 13 in, 2 out]
            n180 = call-poly <userlib>:"DtOLRead.vi"("Number Chan to Read"=w1043, "error in (no error)"=w1044, "Task in"=w1045) -> ("error out"=w1041:errorcluster, "2D Data out"=w1040:dbl[][], "Task out"=w1042:i32)  [unwired: 4 in, 2 out]
            n181 = Index Array(array=w1040, index (row) #1=0 ("index (row)"), index (row) #2=1 ("index (row)"), index (row) #3=2 ("index (row)"), index (row) #4=3 ("index (row)"), index (row) #5=4 ("index (row)")) -> (element #1=w1039:dbl[], element #2=w1033:dbl[], element #3=w1032:dbl[], element #4=w1031:dbl[], element #5=w1030:dbl[])  [unwired: 5 in]
            n182 = Index Array(array=w1030, index=0) -> (element=w1049:dbl)
            n183 = Index Array(array=w1039, index=0) -> (element=w1055:dbl)
            n184 = Index Array(array=w1033, index=0) -> (element=w1060:dbl)
            n185 = Index Array(array=w1032, index=0) -> (element=w1051:dbl)
            n186 = Index Array(array=w1031, index=0) -> (element=w1050:dbl)
            n187 = Bundle("Task out"=w1042, "error out"=w1041) -> (w1052:T8)  [unwired: 1 in]
          }
        }
        n188 = Divide(x=w388, y=u32 1000) -> (x/y=w389:dbl)
        n189 = local read "FILE"() -> (w243:refnum<file>)
        n190 = Build Array (concatenate)(w466, w389) -> (w374:dbl[])
        n191 = property on="TIME GRAPH" class="XYGraph (strict)"("XScale.Mapping Mode"="TIME GRAPH X", "YScale.Mapping Mode"="TIME GRAPH Y") -> ()  [unwired: 2 in, 2 out]
        n192 = property on="MULTIPLE GRAPHS" class="XYGraph (strict)"("XScale.Mapping Mode"="MULTIPLE GRAPHS X", "YScale.Mapping Mode"="MULTIPLE GRAPHS Y") -> ()  [unwired: 2 in, 2 out]
        n193 = Bundle(w376, w296, w297) -> (w249:cluster{dbl, dbl, dbl})  [unwired: 1 in]
        n194 = Unbundle(w249) -> (w293:dbl, w259:dbl, w254:dbl)
        n195 = Unbundle(w249) -> (w191:dbl, w190:dbl, w189:dbl)
        n196 = Multiply(x=w293, y="Current") -> (x*y=w292:dbl)
        n197 = Multiply(x=w254, y="Lock-In, Y") -> (x*y=w255:dbl)
        n198 = Multiply(x=w259, y="Lock-In, X") -> (x*y=w260:dbl)
        n199 = Build Array (concatenate)(w407, w292) -> (w375:dbl[])
        n200 = Build Array (concatenate)(w411, w260) -> (w345:dbl[])
        n201 = Build Array (concatenate)(w410, w255) -> (w344:dbl[])
        n202 = Bundle(w351, w350, w349, w348, w347, "Measurement"=w346) -> (w352:T9)  [unwired: 1 in]
        n203 = Unbundle(w352) -> (w285:dbl, w279:dbl, w274:dbl, w269:dbl, w264:dbl, "Measurement"=w288:dbl)
        n204 = Unbundle(w352) -> (w187:dbl, w186:dbl, w185:dbl, w184:dbl, w183:dbl, "Measurement"=w188:dbl)
        n205 = Format Into String(format string="%08d  %8.2e %12g %14.5e %12.4e %12.4e  %12.4e %12.4e  %12.4e  %12g \\n", initial string=w243, w388, w191, w188, w190, w189, w187, w186, w185, w184, w183) -> ()  [unwired: 1 in, 2 out]
        n206 = Multiply(x=w288, y="2000") -> (x*y=w286:dbl)
        n207 = Multiply(x=w279, y="DAQ A1") -> (x*y=w280:dbl)
        n208 = Multiply(x=w285, y="DAQ A0") -> (x*y=w284:dbl)
        n209 = Multiply(x="DAQ A2", y=w274) -> (x*y=w275:dbl)
        n210 = Multiply(x=w264, y="DAQ A4") -> (x*y=w265:dbl)
        n211 = Multiply(x=w269, y="DAQ A3") -> (x*y=w270:dbl)
        n212 = Build Array (concatenate)(w467, w286) -> (w373:dbl[])
        n213 = Build Array (concatenate)(w379, w284) -> (w372:dbl[])
        n214 = Build Array (concatenate)(w378, w280) -> (w371:dbl[])
        n215 = Build Array (concatenate)(w377, w275) -> (w370:dbl[])
        n216 = Build Array (concatenate)(w457, w270) -> (w369:dbl[])
        n217 = Build Array (concatenate)(w343, w265) -> (w342:dbl[])
        n218 = Bundle(w375, w374, w373, w372, w371, w370, w369, w342, w345, w344) -> (w362:T10)  [unwired: 1 in]
        n219 = Unbundle(w362) -> (w294:dbl[], w252:dbl[], w291:dbl[], w282:dbl[], w277:dbl[], w272:dbl[], w267:dbl[], w261:dbl[], w257:dbl[], w251:dbl[])
        n220 = Bundle(w252, w294) -> (w295:cluster{dbl[], dbl[]})  [unwired: 1 in]
        n221 = Bundle(w252, w291) -> (w290:cluster{dbl[], dbl[]})  [unwired: 1 in]
        n222 = Bundle(w252, w282) -> (w281:cluster{dbl[], dbl[]})  [unwired: 1 in]
        n223 = Bundle(w252, w277) -> (w276:cluster{dbl[], dbl[]})  [unwired: 1 in]
        n224 = Bundle(w252, w267) -> (w266:cluster{dbl[], dbl[]})  [unwired: 1 in]
        n225 = Bundle(w252, w272) -> (w271:cluster{dbl[], dbl[]})  [unwired: 1 in]
        n226 = Bundle(w252, w261) -> (w262:cluster{dbl[], dbl[]})  [unwired: 1 in]
        n227 = Bundle(w252, w257) -> (w256:cluster{dbl[], dbl[]})  [unwired: 1 in]
        n228 = Bundle(w252, w251) -> (w250:cluster{dbl[], dbl[]})  [unwired: 1 in]
        n229 = Build Array(w295, w290, w281, w276, w271, w266, w262, w256, w250) -> (→"TIME GRAPH":cluster{dbl[], dbl[]}[])
        n230 = Unbundle(w362) -> (w361:dbl[], w360:dbl[], w359:dbl[], w358:dbl[], w357:dbl[], w356:dbl[], w355:dbl[], w354:dbl[], w337:dbl[])  [unwired: 1 out]
        n231 = case shown="\"V, Keithley DAQ A3\"" "X-Axis" {
          tunnel: [w487 w529 w564 w592 w634 w669 w704 w729 w764] -> w353
          tunnel: w361 -> [w484 w528 w563 w599 w633 w668 w702 w737 w772]
          tunnel: w360 -> [w501 w519 w562 w598 w632 w667 w701 w736 w771]
          tunnel: w359 -> [w500 w527 w554 w597 w631 w666 w700 w735 w770]
          tunnel: w358 -> [w499 w526 w561 w589 w630 w665 w699 w734 w769]
          tunnel: w357 -> [w498 w525 w560 w596 w624 w664 w698 w733 w768]
          tunnel: w356 -> [w497 w524 w559 w595 w629 w659 w697 w732 w767]
          tunnel: w355 -> [w496 w523 w558 w594 w628 w663 w703 w731 w766]
          tunnel: w354 -> [w495 w522 w557 w593 w627 w662 w696 w738 w765]
          tunnel: w337 -> [w485 w520 w555 w590 w625 w660 w695 w730 w773]
          frame "I, Keithley 6221", Default {
            n232 = Bundle(w484, w501) -> (w494:cluster{dbl[], dbl[]})  [unwired: 1 in]
            n233 = Bundle(w484, w500) -> (w493:cluster{dbl[], dbl[]})  [unwired: 1 in]
            n234 = Bundle(w484, w499) -> (w492:cluster{dbl[], dbl[]})  [unwired: 1 in]
            n235 = Bundle(w484, w498) -> (w491:cluster{dbl[], dbl[]})  [unwired: 1 in]
            n236 = Bundle(w484, w497) -> (w490:cluster{dbl[], dbl[]})  [unwired: 1 in]
            n237 = Bundle(w484, w496) -> (w489:cluster{dbl[], dbl[]})  [unwired: 1 in]
            n238 = Bundle(w484, w495) -> (w488:cluster{dbl[], dbl[]})  [unwired: 1 in]
            n239 = Bundle(w484, w485) -> (w486:cluster{dbl[], dbl[]})  [unwired: 1 in]
            n240 = Build Array(w494, w493, w492, w491, w490, w489, w488, w486) -> (w487:cluster{dbl[], dbl[]}[])
            n241 = property on="MULTIPLE GRAPHS" class="XYGraph (strict)"("XScale.NameLbl.Text"="Keithley 6221, mA" ("X Scale.Name Label.Text")) -> ()  [unwired: 2 in, 2 out]
            n242 = property on="MULTIPLE GRAPHS" class="XYGraph (strict)"("Active Plot"=u32 0, "Plot.Plot Name"="Mult, 2000 V", "Active Plot"=u32 1, "Plot.Plot Name"="DAQ A0", "Active Plot"=u32 2, "Plot.Plot Name"="DAQ A1", "Active Plot"=u32 3, "Plot.Plot Name"="DAQ A2", "Active Plot"=u32 4, "Plot.Plot Name"="DAQ A3", "Active Plot"=u32 5, "Plot.Plot Name"="DAQ A4", "Active Plot"=u32 6, "Plot.Plot Name"="Lock-In, X", "Active Plot"=u32 7, "Plot.Plot Name"="Lock-In, Y") -> ()  [unwired: 2 in, 2 out]
          }
          frame "V, Keithley 2000" {
            n243 = property on="MULTIPLE GRAPHS" class="XYGraph (strict)"("XScale.NameLbl.Text"="Keithley 2000, V" ("X Scale.Name Label.Text")) -> ()  [unwired: 2 in, 2 out]
            n244 = Bundle(w519, w528) -> (w536:cluster{dbl[], dbl[]})  [unwired: 1 in]
            n245 = Bundle(w519, w527) -> (w535:cluster{dbl[], dbl[]})  [unwired: 1 in]
            n246 = Bundle(w519, w526) -> (w534:cluster{dbl[], dbl[]})  [unwired: 1 in]
            n247 = Bundle(w519, w525) -> (w533:cluster{dbl[], dbl[]})  [unwired: 1 in]
            n248 = Bundle(w519, w524) -> (w532:cluster{dbl[], dbl[]})  [unwired: 1 in]
            n249 = Bundle(w519, w523) -> (w531:cluster{dbl[], dbl[]})  [unwired: 1 in]
            n250 = Bundle(w519, w522) -> (w530:cluster{dbl[], dbl[]})  [unwired: 1 in]
            n251 = Bundle(w519, w520) -> (w521:cluster{dbl[], dbl[]})  [unwired: 1 in]
            n252 = Build Array(w536, w535, w534, w533, w532, w531, w530, w521) -> (w529:cluster{dbl[], dbl[]}[])
            n253 = property on="MULTIPLE GRAPHS" class="XYGraph (strict)"("Active Plot"=u32 0, "Plot.Plot Name"="I, 6221 mA", "Active Plot"=u32 1, "Plot.Plot Name"="DAQ A0", "Active Plot"=u32 2, "Plot.Plot Name"="DAQ A1", "Active Plot"=u32 3, "Plot.Plot Name"="DAQ A2", "Active Plot"=u32 4, "Plot.Plot Name"="DAQ A3", "Active Plot"=u32 5, "Plot.Plot Name"="DAQ A4", "Active Plot"=u32 6, "Plot.Plot Name"="Lock-In, X", "Active Plot"=u32 7, "Plot.Plot Name"="Lock-In, Y") -> ()  [unwired: 2 in, 2 out]
          }
          frame "V, Keithley DAQ A0" {
            n254 = property on="MULTIPLE GRAPHS" class="XYGraph (strict)"("XScale.NameLbl.Text"="Keithley DAQ A0, V" ("X Scale.Name Label.Text")) -> ()  [unwired: 2 in, 2 out]
            n255 = Bundle(w554, w555) -> (w556:cluster{dbl[], dbl[]})  [unwired: 1 in]
            n256 = Bundle(w554, w563) -> (w571:cluster{dbl[], dbl[]})  [unwired: 1 in]
            n257 = Bundle(w554, w562) -> (w570:cluster{dbl[], dbl[]})  [unwired: 1 in]
            n258 = Bundle(w554, w561) -> (w569:cluster{dbl[], dbl[]})  [unwired: 1 in]
            n259 = Bundle(w554, w560) -> (w568:cluster{dbl[], dbl[]})  [unwired: 1 in]
            n260 = Bundle(w554, w559) -> (w567:cluster{dbl[], dbl[]})  [unwired: 1 in]
            n261 = Bundle(w554, w558) -> (w566:cluster{dbl[], dbl[]})  [unwired: 1 in]
            n262 = Bundle(w554, w557) -> (w565:cluster{dbl[], dbl[]})  [unwired: 1 in]
            n263 = Build Array(w571, w570, w569, w568, w567, w566, w565, w556) -> (w564:cluster{dbl[], dbl[]}[])
            n264 = property on="MULTIPLE GRAPHS" class="XYGraph (strict)"("Active Plot"=u32 0, "Plot.Plot Name"="I, 6221 mA", "Active Plot"=u32 1, "Plot.Plot Name"="Mult, 2000 V", "Active Plot"=u32 2, "Plot.Plot Name"="DAQ A1", "Active Plot"=u32 3, "Plot.Plot Name"="DAQ A2", "Active Plot"=u32 4, "Plot.Plot Name"="DAQ A3", "Active Plot"=u32 5, "Plot.Plot Name"="DAQ A4", "Active Plot"=u32 6, "Plot.Plot Name"="Lock-In, X", "Active Plot"=u32 7, "Plot.Plot Name"="Lock-In, Y") -> ()  [unwired: 2 in, 2 out]
          }
          frame "V, Keithley DAQ A1" {
            n265 = property on="MULTIPLE GRAPHS" class="XYGraph (strict)"("XScale.NameLbl.Text"="Keithley DAQ A1, V" ("X Scale.Name Label.Text")) -> ()  [unwired: 2 in, 2 out]
            n266 = Bundle(w589, w599) -> (w601:cluster{dbl[], dbl[]})  [unwired: 1 in]
            n267 = Bundle(w589, w598) -> (w602:cluster{dbl[], dbl[]})  [unwired: 1 in]
            n268 = Bundle(w589, w597) -> (w603:cluster{dbl[], dbl[]})  [unwired: 1 in]
            n269 = Bundle(w589, w596) -> (w604:cluster{dbl[], dbl[]})  [unwired: 1 in]
            n270 = Bundle(w589, w595) -> (w605:cluster{dbl[], dbl[]})  [unwired: 1 in]
            n271 = Bundle(w589, w594) -> (w606:cluster{dbl[], dbl[]})  [unwired: 1 in]
            n272 = Bundle(w589, w593) -> (w607:cluster{dbl[], dbl[]})  [unwired: 1 in]
            n273 = Bundle(w589, w590) -> (w591:cluster{dbl[], dbl[]})  [unwired: 1 in]
            n274 = Build Array(w601, w602, w603, w604, w605, w606, w607, w591) -> (w592:cluster{dbl[], dbl[]}[])
            n275 = property on="MULTIPLE GRAPHS" class="XYGraph (strict)"("Active Plot"=u32 0, "Plot.Plot Name"="I, 6221 mA", "Active Plot"=u32 1, "Plot.Plot Name"="Mult, 2000 V", "Active Plot"=u32 2, "Plot.Plot Name"="DAQ A0", "Active Plot"=u32 3, "Plot.Plot Name"="DAQ A2", "Active Plot"=u32 4, "Plot.Plot Name"="DAQ A3", "Active Plot"=u32 5, "Plot.Plot Name"="DAQ A4", "Active Plot"=u32 6, "Plot.Plot Name"="Lock-In, X", "Active Plot"=u32 7, "Plot.Plot Name"="Lock-In, Y") -> ()  [unwired: 2 in, 2 out]
          }
          frame "V, Keithley DAQ A2" {
            n276 = property on="MULTIPLE GRAPHS" class="XYGraph (strict)"("XScale.NameLbl.Text"="Keithley DAQ A2, V" ("X Scale.Name Label.Text")) -> ()  [unwired: 2 in, 2 out]
            n277 = Bundle(w624, w633) -> (w635:cluster{dbl[], dbl[]})  [unwired: 1 in]
            n278 = Bundle(w624, w632) -> (w636:cluster{dbl[], dbl[]})  [unwired: 1 in]
            n279 = Bundle(w624, w631) -> (w637:cluster{dbl[], dbl[]})  [unwired: 1 in]
            n280 = Bundle(w624, w630) -> (w638:cluster{dbl[], dbl[]})  [unwired: 1 in]
            n281 = Bundle(w624, w629) -> (w639:cluster{dbl[], dbl[]})  [unwired: 1 in]
            n282 = Bundle(w624, w628) -> (w640:cluster{dbl[], dbl[]})  [unwired: 1 in]
            n283 = Bundle(w624, w627) -> (w641:cluster{dbl[], dbl[]})  [unwired: 1 in]
            n284 = Bundle(w624, w625) -> (w626:cluster{dbl[], dbl[]})  [unwired: 1 in]
            n285 = Build Array(w635, w636, w637, w638, w639, w640, w641, w626) -> (w634:cluster{dbl[], dbl[]}[])
            n286 = property on="MULTIPLE GRAPHS" class="XYGraph (strict)"("Active Plot"=u32 0, "Plot.Plot Name"="I, 6221 mA", "Active Plot"=u32 1, "Plot.Plot Name"="Mult, 2000 V", "Active Plot"=u32 2, "Plot.Plot Name"="DAQ A0", "Active Plot"=u32 3, "Plot.Plot Name"="DAQ A1", "Active Plot"=u32 4, "Plot.Plot Name"="DAQ A3", "Active Plot"=u32 5, "Plot.Plot Name"="DAQ A4", "Active Plot"=u32 6, "Plot.Plot Name"="Lock-In, X", "Active Plot"=u32 7, "Plot.Plot Name"="Lock-In, Y") -> ()  [unwired: 2 in, 2 out]
          }
          frame "V, Keithley DAQ A3" {
            n287 = property on="MULTIPLE GRAPHS" class="XYGraph (strict)"("XScale.NameLbl.Text"="Keithley DAQ A3, V" ("X Scale.Name Label.Text")) -> ()  [unwired: 2 in, 2 out]
            n288 = Bundle(w659, w668) -> (w670:cluster{dbl[], dbl[]})  [unwired: 1 in]
            n289 = Bundle(w659, w667) -> (w671:cluster{dbl[], dbl[]})  [unwired: 1 in]
            n290 = Bundle(w659, w666) -> (w672:cluster{dbl[], dbl[]})  [unwired: 1 in]
            n291 = Bundle(w659, w665) -> (w673:cluster{dbl[], dbl[]})  [unwired: 1 in]
            n292 = Bundle(w659, w664) -> (w674:cluster{dbl[], dbl[]})  [unwired: 1 in]
            n293 = Bundle(w659, w663) -> (w675:cluster{dbl[], dbl[]})  [unwired: 1 in]
            n294 = Bundle(w659, w662) -> (w676:cluster{dbl[], dbl[]})  [unwired: 1 in]
            n295 = Bundle(w659, w660) -> (w661:cluster{dbl[], dbl[]})  [unwired: 1 in]
            n296 = Build Array(w670, w671, w672, w673, w674, w675, w676, w661) -> (w669:cluster{dbl[], dbl[]}[])
            n297 = property on="MULTIPLE GRAPHS" class="XYGraph (strict)"("Active Plot"=u32 0, "Plot.Plot Name"="I, 6221 mA", "Active Plot"=u32 1, "Plot.Plot Name"="Mult, 2000 V", "Active Plot"=u32 2, "Plot.Plot Name"="DAQ A0", "Active Plot"=u32 3, "Plot.Plot Name"="DAQ A1", "Active Plot"=u32 4, "Plot.Plot Name"="DAQ A2", "Active Plot"=u32 5, "Plot.Plot Name"="DAQ A4", "Active Plot"=u32 6, "Plot.Plot Name"="Lock-In, X", "Active Plot"=u32 7, "Plot.Plot Name"="Lock-In,Y") -> ()  [unwired: 2 in, 2 out]
          }
          frame "V, Keithley DAQ A4" {
            n298 = property on="MULTIPLE GRAPHS" class="XYGraph (strict)"("XScale.NameLbl.Text"="Keithley DAQ A4, V" ("X Scale.Name Label.Text")) -> ()  [unwired: 2 in, 2 out]
            n299 = Bundle(w703, w702) -> (w706:cluster{dbl[], dbl[]})  [unwired: 1 in]
            n300 = Bundle(w703, w701) -> (w707:cluster{dbl[], dbl[]})  [unwired: 1 in]
            n301 = Bundle(w703, w700) -> (w708:cluster{dbl[], dbl[]})  [unwired: 1 in]
            n302 = Bundle(w703, w699) -> (w709:cluster{dbl[], dbl[]})  [unwired: 1 in]
            n303 = Bundle(w703, w698) -> (w710:cluster{dbl[], dbl[]})  [unwired: 1 in]
            n304 = Bundle(w703, w697) -> (w711:cluster{dbl[], dbl[]})  [unwired: 1 in]
            n305 = Bundle(w703, w696) -> (w712:cluster{dbl[], dbl[]})  [unwired: 1 in]
            n306 = Bundle(w703, w695) -> (w705:cluster{dbl[], dbl[]})  [unwired: 1 in]
            n307 = Build Array(w706, w707, w708, w709, w710, w711, w712, w705) -> (w704:cluster{dbl[], dbl[]}[])
            n308 = property on="MULTIPLE GRAPHS" class="XYGraph (strict)"("Active Plot"=u32 0, "Plot.Plot Name"="I, 6221 mA", "Active Plot"=u32 1, "Plot.Plot Name"="Mult, 2000 V", "Active Plot"=u32 2, "Plot.Plot Name"="DAQ A0", "Active Plot"=u32 3, "Plot.Plot Name"="DAQ A1", "Active Plot"=u32 4, "Plot.Plot Name"="DAQ A2", "Active Plot"=u32 5, "Plot.Plot Name"="DAQ A3", "Active Plot"=u32 6, "Plot.Plot Name"="Lock-In, X", "Active Plot"=u32 7, "Plot.Plot Name"="Lock-In, Y") -> ()  [unwired: 2 in, 2 out]
          }
          frame "V, Lock-In X" {
            n309 = property on="MULTIPLE GRAPHS" class="XYGraph (strict)"("XScale.NameLbl.Text"="Lock-In X, V" ("X Scale.Name Label.Text")) -> ()  [unwired: 2 in, 2 out]
            n310 = Bundle(w738, w737) -> (w740:cluster{dbl[], dbl[]})  [unwired: 1 in]
            n311 = Bundle(w738, w736) -> (w741:cluster{dbl[], dbl[]})  [unwired: 1 in]
            n312 = Bundle(w738, w735) -> (w742:cluster{dbl[], dbl[]})  [unwired: 1 in]
            n313 = Bundle(w738, w734) -> (w743:cluster{dbl[], dbl[]})  [unwired: 1 in]
            n314 = Bundle(w738, w733) -> (w744:cluster{dbl[], dbl[]})  [unwired: 1 in]
            n315 = Bundle(w738, w732) -> (w745:cluster{dbl[], dbl[]})  [unwired: 1 in]
            n316 = Bundle(w738, w731) -> (w746:cluster{dbl[], dbl[]})  [unwired: 1 in]
            n317 = Bundle(w738, w730) -> (w739:cluster{dbl[], dbl[]})  [unwired: 1 in]
            n318 = Build Array(w740, w741, w742, w743, w744, w745, w746, w739) -> (w729:cluster{dbl[], dbl[]}[])
            n319 = property on="MULTIPLE GRAPHS" class="XYGraph (strict)"("Active Plot"=u32 0, "Plot.Plot Name"="I, 6221 mA", "Active Plot"=u32 1, "Plot.Plot Name"="Mult, 2000 V", "Active Plot"=u32 2, "Plot.Plot Name"="DAQ A0", "Active Plot"=u32 3, "Plot.Plot Name"="DAQ A1", "Active Plot"=u32 4, "Plot.Plot Name"="DAQ A2", "Active Plot"=u32 5, "Plot.Plot Name"="DAQ A3", "Active Plot"=u32 6, "Plot.Plot Name"="DAQ A4", "Active Plot"=u32 7, "Plot.Plot Name"="Lock-In, Y") -> ()  [unwired: 2 in, 2 out]
          }
          frame "V, Lock-In Y" {
            n320 = property on="MULTIPLE GRAPHS" class="XYGraph (strict)"("XScale.NameLbl.Text"="Lock-In Y, V" ("X Scale.Name Label.Text")) -> ()  [unwired: 2 in, 2 out]
            n321 = Bundle(w773, w772) -> (w781:cluster{dbl[], dbl[]})  [unwired: 1 in]
            n322 = Bundle(w773, w771) -> (w780:cluster{dbl[], dbl[]})  [unwired: 1 in]
            n323 = Bundle(w773, w770) -> (w779:cluster{dbl[], dbl[]})  [unwired: 1 in]
            n324 = Bundle(w773, w769) -> (w778:cluster{dbl[], dbl[]})  [unwired: 1 in]
            n325 = Bundle(w773, w768) -> (w777:cluster{dbl[], dbl[]})  [unwired: 1 in]
            n326 = Bundle(w773, w767) -> (w776:cluster{dbl[], dbl[]})  [unwired: 1 in]
            n327 = Bundle(w773, w766) -> (w775:cluster{dbl[], dbl[]})  [unwired: 1 in]
            n328 = Bundle(w773, w765) -> (w774:cluster{dbl[], dbl[]})  [unwired: 1 in]
            n329 = Build Array(w781, w780, w779, w778, w777, w776, w775, w774) -> (w764:cluster{dbl[], dbl[]}[])
            n330 = property on="MULTIPLE GRAPHS" class="XYGraph (strict)"("Active Plot"=u32 0, "Plot.Plot Name"="I, 6221 mA", "Active Plot"=u32 1, "Plot.Plot Name"="Mult, 2000 V", "Active Plot"=u32 2, "Plot.Plot Name"="DAQ A0", "Active Plot"=u32 3, "Plot.Plot Name"="DAQ A1", "Active Plot"=u32 4, "Plot.Plot Name"="DAQ A2", "Active Plot"=u32 5, "Plot.Plot Name"="DAQ A3", "Active Plot"=u32 6, "Plot.Plot Name"="DAQ A4", "Active Plot"=u32 7, "Plot.Plot Name"="Lock-In, X") -> ()  [unwired: 2 in, 2 out]
          }
        }
        "MULTIPLE GRAPHS" <- w353
        n331 = Unbundle(w362) -> (w368:dbl[], w367:dbl[], w366:dbl[], w365:dbl[], w364:dbl[], w363:dbl[], w338:dbl[], w339:dbl[], w340:dbl[], w341:dbl[])
        n332 = Multiply(x="Time Delay", y=u16 1000) -> (x*y=w242:u16)
        n333 = Wait Until Next ms Multiple(millisecond multiple=w242) -> ()  [unwired: 1 out]
        "2000" <- w450
        "DAQ A0" <- w351
        "DAQ A1" <- w350
        "DAQ A2" <- w349
        "DAQ A3" <- w348
        "DAQ A4" <- w347
      }
    }
    frame #3 {
      # "Closing instrumental \nconnections"
      n334 = flat-sequence {
        frame #0 {
          w1072 = TRUE ("Visible")
          n335 = property on="Slope" class="Ring (strict)"("Visible"=w1072) -> ()  [unwired: 2 in, 2 out]
          n336 = property on="Range" class="Ring (strict)"("Visible"=w1072) -> ()  [unwired: 2 in, 2 out]
          n337 = property on="Time Constant" class="Ring (strict)"("Visible"=w1072) -> ()  [unwired: 2 in, 2 out]
          n338 = property on="Dynamic Reserve" class="Ring (strict)"("Visible"=w1072) -> ()  [unwired: 2 in, 2 out]
          n339 = property on="Auto Sensitivity" class="Bool (strict)"("Visible"=w1072) -> ()  [unwired: 2 in, 2 out]
          n340 = property on="Auto Measure" class="Bool (strict)"("Visible"=w1072) -> ()  [unwired: 2 in, 2 out]
        }
        frame #1 {
          w1073 = TRUE ("Visible")
          n341 = property on="Start \ncurrent (A)" class="DigNum (strict)"("Visible"=w1073) -> ()  [unwired: 2 in, 2 out]
          n342 = property on="Stop\ncurrent (A)" class="DigNum (strict)"("Visible"=w1073) -> ()  [unwired: 2 in, 2 out]
          n343 = property on="LIMIT" class="Bool (strict)"("Visible"=w1073) -> ()  [unwired: 2 in, 2 out]
          n344 = property on="LIMIT" class="Bool (strict)"("Visible"=w1073) -> ()  [unwired: 2 in, 2 out]
          n345 = property on="Start cur prefix" class="Ring (strict)"("Visible"=w1073) -> ()  [unwired: 2 in, 2 out]
          n346 = property on="Stop cur prefix" class="Ring (strict)"("Visible"=w1073) -> ()  [unwired: 2 in, 2 out]
          n347 = property on="Step  (A)" class="DigNum (strict)"("Visible"=w1073) -> ()  [unwired: 2 in, 2 out]
          n348 = property on="Number \nof points" class="DigNum (strict)"("Visible"=w1073) -> ()  [unwired: 2 in, 2 out]
          n349 = property on="Time Delay" class="Ring (strict)"("Visible"=w1073) -> ()  [unwired: 2 in, 2 out]
          n350 = property on="Error Code" class="Str"("Visible"=w1073) -> ()  [unwired: 2 in, 2 out]
        }
      }
      n351 = Unbundle(w1064) -> ("Task out"=w1063:i32, "error out"=w1062:errorcluster)
      n352 = call <instrlib>:"Close.vi"("VISA resource name"=w1069, "error in (no error)"=w1070) -> ()  [unwired: 17 in, 1 out]
      n353 = call "SR51XX Close"("error in (no error)"=w1065, "VISA session"=w1066) -> ()  [unwired: 1 out]
      n354 = call <instrlib>:"Close.vi"("VISA resource name"=w1067, "error in (no error)"=w1068) -> ()  [unwired: 13 in, 1 out]
      n355 = call <userlib>:"DtOLCloseTask.vi"("Error in"=w1062, "Task in"=w1063) -> ("Error Out"=w1071:errorcluster)  [unwired: 9 in]
      n356 = call <vilib>:"Simple Error Handler.vi"("error in (no error)"=w1071) -> ()  [unwired: 4 in, 5 out]
    }
  }
